vi "seq scan current(SubVI).vi"(6 "字符串":string, 9 "queue out 2":refnum<queue>, 10 "queue out":refnum<queue>) -> (0 "错误输出":errorcluster)   [LabVIEW 2019, in "Take Seq.lvlib"]
uses:
  Take Seq.lvlib
  error.ctl
  lib/QDInstrument.dll
  SubVI.lvlib
panel:
  # "(真是通道1，假是通道2)"
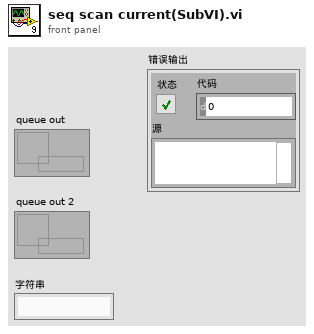
[diagram p1: front panel]
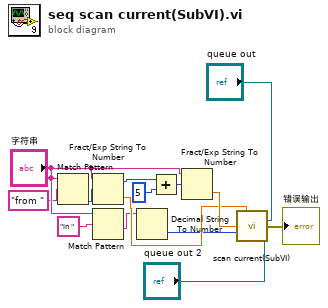
[diagram p0: block diagram]
diagram:
  n1 = Match Pattern(string="字符串", regular expression="from " ("正则表达式")) -> (offset past match=w4:i32)  [unwired: 1 in, 3 out]
  n2 = Fract/Exp String To Number(string="字符串", offset=w4) -> (offset past number=w6:i32, number=w11:dbl)  [unwired: 2 in]
  n3 = Match Pattern(string="字符串", regular expression="in " ("正则表达式")) -> (after substring=w9:string)  [unwired: 1 in, 3 out]
  n4 = Decimal String To Number(string=w9) -> (number=w10:i32)  [unwired: 2 in, 1 out]
  n5 = Add(x=w6, y=5) -> (x+y=w5:i32)
  n6 = Fract/Exp String To Number(string="字符串", offset=w5) -> (number=w12:dbl)  [unwired: 2 in, 1 out]
  n7 = call "scan current(SubVI).vi"("Current"=w11, "data"="queue out", "Current 2"=w12, "steps number"=w10, "config"="queue out 2") -> ("错误输出"=→"错误输出":errorcluster)  [unwired: 10 in]
